vi "PXI-Set Stop Condition.vi"(0 "Stop on Max Presentations?":bool=TRUE, 5 "Number of presentations":i32, 11 "error in (no error)":errorcluster) -> (15 "error out":errorcluster)   [LabVIEW 2020]
uses:
  DAQ Engine VIs/PXI Globals.vi
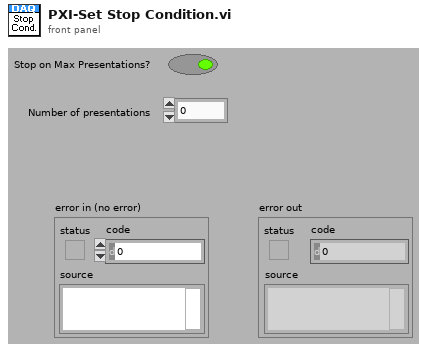
[diagram p1: front panel]
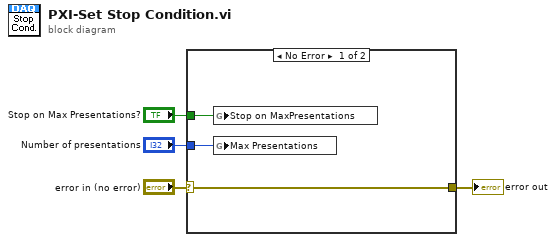
[diagram p0: block diagram]
diagram:
  n1 = case shown="No Error" "error in (no error)" {
    selector: "error in (no error)" -> [w5 w8]
    tunnel: "Stop on Max Presentations?" -> [w7 _]
    tunnel: "Number of presentations" -> [w6 _]
    tunnel: [w5 w8] -> w1
    frame No Error {
      n2 = global write "PXI Globals.vi" "Stop on MaxPresentations"(w7) -> ()
      n3 = global write "PXI Globals.vi" "Max Presentations"(w6) -> ()
    }
    frame Error {
    }
  }
  "error out" <- w1
